vi "Error Handler.vi"() -> ()   [LabVIEW 2015]
uses:
  <vilib>/ErrorRing/Error Ring.xnode
panel:
  out "Signal > 75 % 2":bool
  out "Signal > 50 % 2":bool
  out "Signal > 25% 2":bool
  out "Signal > 0% 2":bool
  out "Battery > 75 % 2":bool
  out "Battery > 50 % 2":bool
  out "Battery > 25% 2":bool
  out "Battery > 0% 2":bool
  out "timed out?\nSignal potentiometer":bool
  out "Signal > 75 %":bool
  out "Signal > 50 %":bool
  out "Signal > 25%":bool
  out "Signal > 0%":bool
  out "Battery > 75 %":bool
  out "Battery > 50 %":bool
  out "Battery > 25%":bool
  out "Battery > 0%":bool
  out "timed out?\nBattery potentiometer":bool
  out "timed out?\nBattery Thermometer":bool
  out "timed out?\nLink Quality\nThermometer":bool
  out "Low radio signal\nfor potentiometer":errorcluster
  out "Low Battery\nfor potentiometer":errorcluster
  out "No Signal \non thermometer":errorcluster
  in  "stop":bool
  out "No Signal\non potentiometer":errorcluster
  in  "stop":bool
  out "Low radio signal\nfor thermometer":errorcluster
  out "Low Battery\nfor thermometer":errorcluster
  # "Battery potentiometer"
  # "Signal quality potentiometer"
  # "Battery Thermometer"
  # "Signal Thermometer"
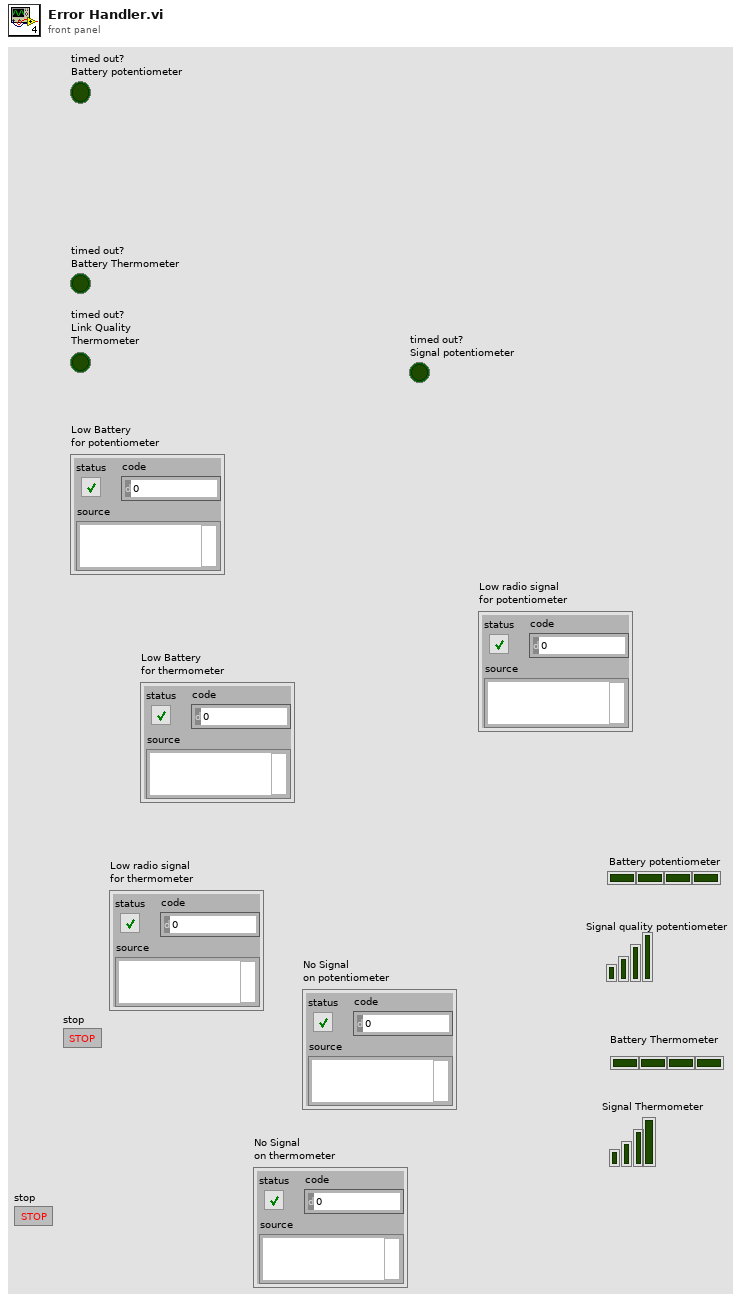
[diagram p1: front panel]
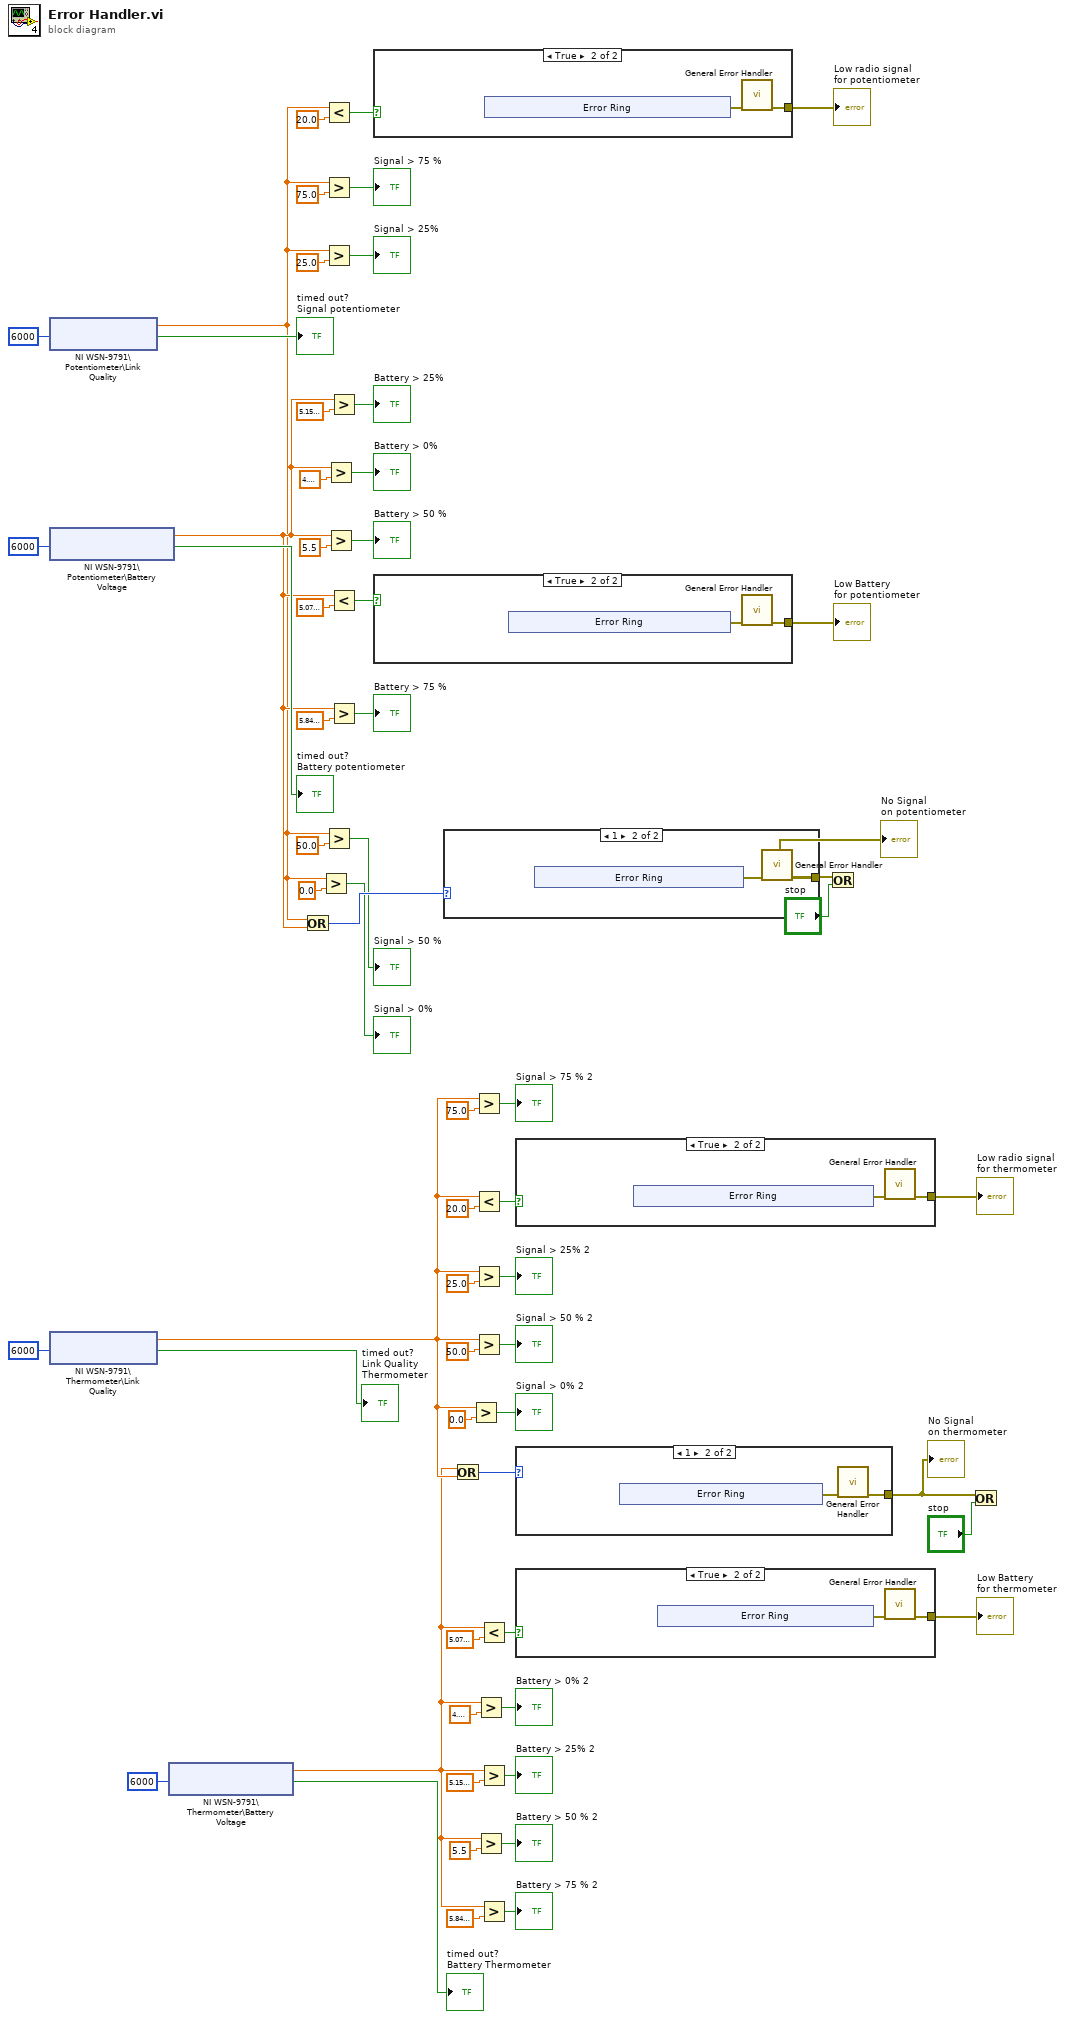
[diagram p0: block diagram]
diagram:
  n1 = shared-variable "NI WSN-9791\\Potentiometer\\Link Quality"(6000 ("ms timeout (0)")) -> (w3:sgl, →"timed out?\nSignal potentiometer":bool)  [unwired: 1 in, 1 out]
  n2 = shared-variable "NI WSN-9791\\Potentiometer\\Battery Voltage"(6000 ("ms timeout (0)")) -> (w4:sgl, →"timed out?\nBattery potentiometer":bool)  [unwired: 1 in, 1 out]
  n3 = shared-variable "NI WSN-9791\\Thermometer\\Link Quality"(6000 ("ms timeout (0)")) -> (w2:sgl, →"timed out?\nLink Quality\nThermometer":bool)  [unwired: 1 in, 1 out]
  n4 = shared-variable "NI WSN-9791\\Thermometer\\Battery Voltage"(6000 ("ms timeout (0)")) -> (w1:sgl, →"timed out?\nBattery Thermometer":bool)  [unwired: 1 in, 1 out]
  n5 = Or(x=w3, y=w4) -> (x .or. y?=w58:i32)
  n6 = Greater?(x=w3, y=sgl 0.0) -> (0:→"Signal > 0%":bool)
  n7 = Less?(x=w3, y=sgl 20.0) -> (x < y?=w29:bool)
  n8 = Greater?(x=w3, y=sgl 75.0) -> (0:→"Signal > 75 %":bool)
  n9 = Greater?(x=w3, y=sgl 25.0) -> (0:→"Signal > 25%":bool)
  n10 = Greater?(x=w3, y=sgl 50.0) -> (0:→"Signal > 50 %":bool)
  n11 = Greater?(x=w4, y=sgl 4.8) -> (0:→"Battery > 0%":bool)
  n12 = Greater?(x=w4, y=sgl 5.5) -> (0:→"Battery > 50 %":bool)
  n13 = Greater?(x=w4, y=sgl 5.15) -> (0:→"Battery > 25%":bool)
  n14 = Less?(x=w4, y=sgl 5.08) -> (x < y?=w49:bool)
  n15 = Greater?(x=w4, y=sgl 5.85) -> (0:→"Battery > 75 %":bool)
  n16 = case shown="True" w29 {
    tunnel: [_ w64] -> w53
    frame False {
    }
    frame True {
      n17 = xnode "Error Ring"() -> ("error out"=w63:errorcluster)
      n18 = call <vilib>:"General Error Handler.vi"("error in (no error)"=w63) -> ("error out"=w64:errorcluster)  [unwired: 10 in, 4 out]
    }
  }
  "Low radio signal\nfor potentiometer" <- w53
  n19 = case shown="True" w49 {
    tunnel: [_ w67] -> w54
    frame False {
    }
    frame True {
      n20 = xnode "Error Ring"() -> ("error out"=w66:errorcluster)
      n21 = call <vilib>:"General Error Handler.vi"("error in (no error)"=w66) -> ("error out"=w67:errorcluster)  [unwired: 10 in, 4 out]
    }
  }
  "Low Battery\nfor potentiometer" <- w54
  n22 = case shown="1" w58 {
    tunnel: [_ w70] -> w59
    frame 0, Default {
    }
    frame 1 {
      n23 = xnode "Error Ring"() -> ("error out"=w69:errorcluster)
      n24 = call <vilib>:"General Error Handler.vi"("error in (no error)"=w69) -> ("error out"=w70:errorcluster)  [unwired: 10 in, 4 out]
    }
  }
  "No Signal\non potentiometer" <- w59
  n25 = Or(x=w1, y=w2) -> (x .or. y?=w55:i32)
  n26 = Greater?(x=w2, y=sgl 0.0) -> (0:→"Signal > 0% 2":bool)
  n27 = Greater?(x=w2, y=sgl 75.0) -> (0:→"Signal > 75 % 2":bool)
  n28 = Less?(x=w2, y=sgl 20.0) -> (x < y?=w10:bool)
  n29 = Greater?(x=w2, y=sgl 25.0) -> (0:→"Signal > 25% 2":bool)
  n30 = Greater?(x=w2, y=sgl 50.0) -> (0:→"Signal > 50 % 2":bool)
  n31 = Greater?(x=w1, y=sgl 4.8) -> (0:→"Battery > 0% 2":bool)
  n32 = Greater?(x=w1, y=sgl 5.5) -> (0:→"Battery > 50 % 2":bool)
  n33 = Less?(x=w1, y=sgl 5.08) -> (x < y?=w5:bool)
  n34 = Greater?(x=w1, y=sgl 5.15) -> (0:→"Battery > 25% 2":bool)
  n35 = Greater?(x=w1, y=sgl 5.85) -> (0:→"Battery > 75 % 2":bool)
  n36 = case shown="True" w10 {
    tunnel: [_ w73] -> w61
    frame False {
    }
    frame True {
      n37 = xnode "Error Ring"() -> ("error out"=w72:errorcluster)
      n38 = call <vilib>:"General Error Handler.vi"("error in (no error)"=w72) -> ("error out"=w73:errorcluster)  [unwired: 10 in, 4 out]
    }
  }
  "Low radio signal\nfor thermometer" <- w61
  n39 = case shown="1" w55 {
    tunnel: [_ w76] -> w56
    frame 0, Default {
    }
    frame 1 {
      n40 = xnode "Error Ring"() -> ("error out"=w75:errorcluster)
      n41 = call <vilib>:"General Error Handler.vi"("error in (no error)"=w75) -> ("error out"=w76:errorcluster)  [unwired: 10 in, 4 out]
    }
  }
  "No Signal \non thermometer" <- w56
  n42 = case shown="True" w5 {
    tunnel: [_ w79] -> w62
    frame False {
    }
    frame True {
      n43 = xnode "Error Ring"() -> ("error out"=w78:errorcluster)
      n44 = call <vilib>:"General Error Handler.vi"("error in (no error)"=w78) -> ("error out"=w79:errorcluster)  [unwired: 10 in, 4 out]
    }
  }
  "Low Battery\nfor thermometer" <- w62
  n45 = Or(x=w59, y="stop") -> ()  [unwired: 1 out]
  n46 = Or(x=w56, y="stop") -> ()  [unwired: 1 out]
